vi "Intent.vi"(1 "Purity":bool, 2 "Sin":bool) -> (0 "The Truth":bool)   [LabVIEW 2013]
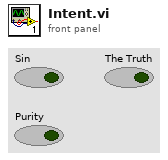
[diagram p1: front panel]
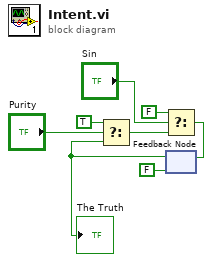
[diagram p0: block diagram]
diagram:
  n1 = feedback #1(FALSE ("Pressed? Array[4]")) -> (w8:bool)
  "The Truth" <- w8
  n2 = Select(t=TRUE, s="Purity", f=w8) -> (s? t:f=w4:bool)
  n3 = Select(t=FALSE, s="Sin", f=w4) -> (s? t:f=w2:bool)
  n4 = feedback-in #1(w2) -> ()
